vi "rethinkdb_msg_error.vi"(8 "error in (no error)":errorcluster, 11 "message":string) -> (0 "error out":errorcluster, 3 "error":errorcluster)   [LabVIEW 2017]
uses:
  cabca6b0-f2c7-43cf-a6e5-c7a1e05d8cdf.vi
  json/rethinkdb_json_to_cluster.vi
  json/rethinkdb_json_type_cast.vi
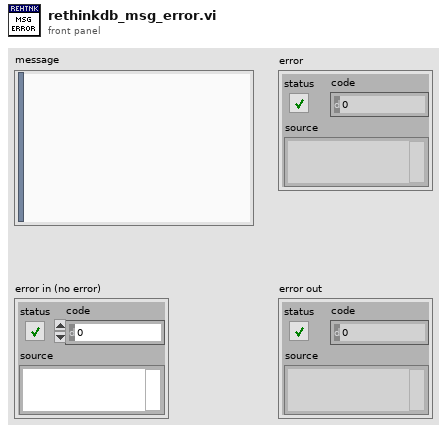
[diagram p1: front panel]
types:
  T1 = cluster{"error_code":i32, "error":string, "success":bool}
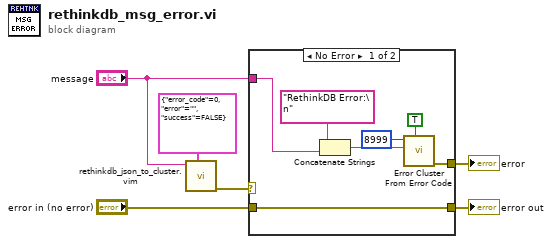
[diagram p0: block diagram]
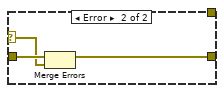
[diagram p2: hidden frame]
diagram:
  n1 = call "rethinkdb_json_to_cluster.vim"("type"=T1 {"error_code"=0, "error"="", "success"=FALSE} ("handshake"), "json"="message") -> ("error out"=w1:errorcluster)  [unwired: 7 in, 2 out]
  n2 = case shown="No Error" w1 {
    selector: w1 -> [_ w14]
    tunnel: "message" -> [w13 _]
    tunnel: [w8 w15] -> w6
    tunnel: [w7 _] -> w3
    tunnel: "error in (no error)" -> [w8 w16]
    frame No Error {
      n3 = Concatenate Strings("RethinkDB Error:\n" ("error message (\"\")"), w13) -> (w9:string)
      n4 = call <vilib>:"Error Cluster From Error Code.vi"("show call chain? (False)"=TRUE, "error message (\"\")"=w9, "error code (0)"=8999) -> ("error out"=w7:errorcluster)  [unwired: 6 in]
    }
    frame Error {
      n5 = Merge Errors(w16, w14) -> (w15:errorcluster)
    }
  }
  "error out" <- w6
  "error" <- w3
